vi "AstarFindPath.vi"(8 "error in (no error)":errorcluster, 9 "goal node":cluster{"X":i32, "Y":i32}={"X"=32, "Y"=32}, 10 "start node":cluster{"X":i32, "Y":i32}={"X"=3, "Y"=3}, 11 "map reference in":refnum<data-value>) -> (0 "error out":errorcluster, 1 "Planned Path":cluster{i32[], i32[]}, 2 "intensity values":dbl[][](array[numeric]), 3 "map reference out":refnum<data-value>)   [LabVIEW 2019]
uses:
  <vilib>/robotics/Navigation/shared/WorldMap/OccupancyGridWorldMap/NI_Robotics_OccupancyGridWorldMap.lvclass
  C:/Program Files (x86)/National Instruments/LabVIEW 2019/vi.lib/robotics/Navigation/shared/WorldMap/AbstractWorldMap/NI_Robotics_AbstractWorldMap.lvclass
  <vilib>/robotics/Navigation/shared/MapNode/OccupancyGridNode/NI_Robotics_OccupancyGridMapNode.lvclass
  C:/Program Files (x86)/National Instruments/LabVIEW 2019/vi.lib/robotics/Navigation/shared/MapNode/AbstractAstarNode/NI_Robotics_AbstractAstarNode.lvclass
  <vilib>/robotics/Navigation/NI_Robotics_Navigation .lvlib
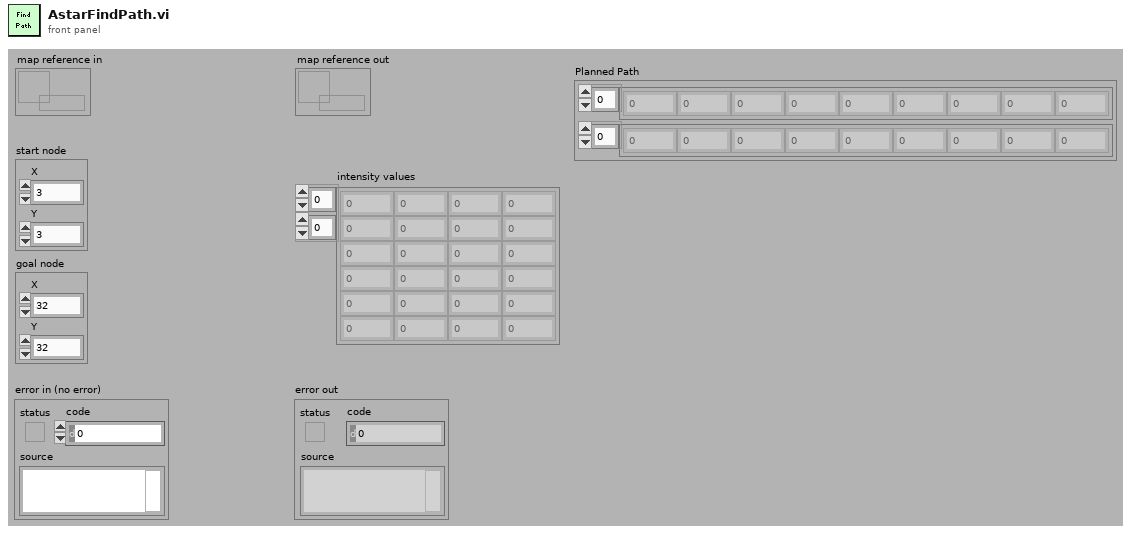
[diagram p1: front panel]
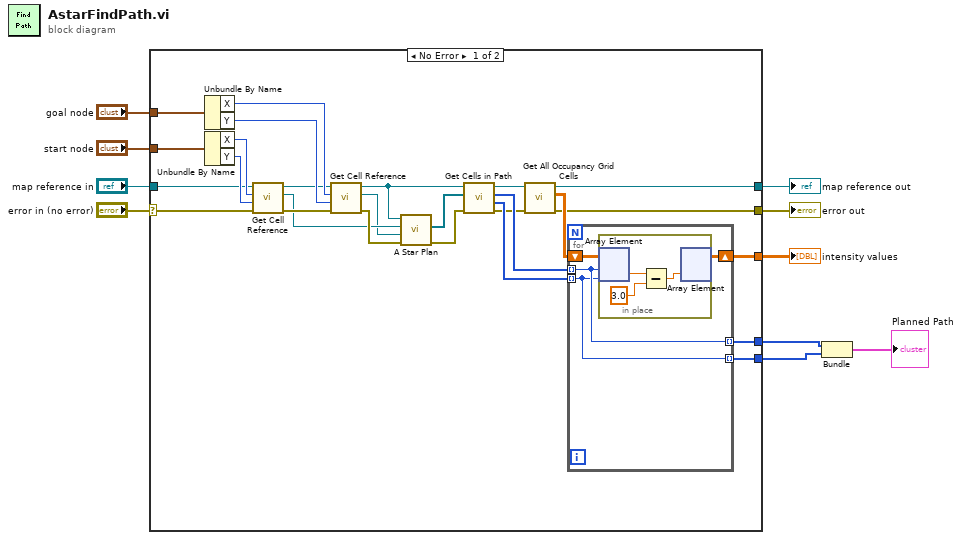
[diagram p0: block diagram]
diagram:
  n1 = case shown="No Error" "error in (no error)" {
    selector: "error in (no error)" -> [w18 w44]
    tunnel: "map reference in" -> [w19 w45]
    tunnel: "goal node" -> [w17 _]
    tunnel: "start node" -> [w16 _]
    tunnel: [w15 _] -> w6
    tunnel: [w14 w45] -> w5
    tunnel: [w13 w44] -> w4
    tunnel: [w12 _] -> w3
    tunnel: [w11 _] -> w2
    frame No Error {
      n2 = Unbundle By Name(w17) -> ("X"=w35:i32, "Y"=w36:i32)
      n3 = Unbundle By Name(w16) -> ("X"=w33:i32, "Y"=w34:i32)
      n4 = call <vilib>:"Get Cell Reference.vi"("error in (no error)"=w18, "y"=w34, "x"=w33, "map reference in"=w19) -> ("error out"=w23:errorcluster, "cell reference"=w21:refnum<data-value>, "map reference out"=w27:refnum<data-value>)  [unwired: 4 in, 1 out]
      n5 = call <vilib>:"Get Cell Reference.vi"("error in (no error)"=w23, "y"=w36, "x"=w35, "map reference in"=w27) -> ("error out"=w28:errorcluster, "cell reference"=w20:refnum<data-value>, "map reference out"=w25:refnum<data-value>)  [unwired: 4 in, 1 out]
      n6 = call <vilib>:"A Star Plan.vi"("error in (no error)"=w28, "goal reference"=w20, "start reference"=w21, "map reference in"=w25) -> ("error out"=w29:errorcluster, "path references"=w26:refnum<data-value>[])  [unwired: 4 in, 2 out]
      n7 = call <vilib>:"Get Cells in Path.vi"("error in (no error)"=w29, "path references"=w26, "map reference in"=w25) -> ("error out"=w22:errorcluster, "y coordinates"=w32:i32[], "x coordinates"=w31:i32[], "map reference out"=w24:refnum<data-value>)  [unwired: 5 in]
      n8 = call <vilib>:"Get All Occupancy Grid Cells.vi"("error in (no error)"=w22, "map reference in"=w24) -> ("error out"=w13:errorcluster, "occupancy grid"=w30:dbl[][], "map reference out"=w14:refnum<data-value>)  [unwired: 7 in]
      n9 = for {
        tunnel: w32 -> [w37] mode=indexing
        tunnel: w31 -> [w38] mode=indexing
        shift-right: [w39] -> w15
        shift-left: w30 -> [w40]
        tunnel: [w38] -> w12 mode=indexing
        tunnel: [w37] -> w11 mode=indexing
        n10 = in-place {
          n11 = in-place-array #1(w40, w38, w37) -> (w42:dbl)
          n12 = Subtract(x=w42, y=3.0) -> (x-y=w41:dbl)
          n13 = in-place-array #1(w41) -> (w39:dbl[][])  [unwired: 2 out]
        }
      }
    }
    frame Error {
    }
  }
  "error out" <- w4
  "intensity values" <- w6
  "map reference out" <- w5
  n14 = Bundle(w3, w2) -> (→"Planned Path":cluster{i32[], i32[]})  [unwired: 1 in]
